vi "ATF RIg Graphs V1.1.vi"() -> ()   [LabVIEW 2022 SP3]
uses:
  Source code/Globals/ATF1_ACQ.vi
  Source code/Globals/Main_global.vi
panel:
  out "?":waveform(dbl)[](graph)
  out "?":cluster{dbl, dbl, dbl, dbl, dbl, dbl}(graph)
  out "?":waveform(dbl)[](graph)
  out "?":T1(graph)
  out "?":waveform(dbl)[](graph)
  out "?":cluster{dbl, dbl, dbl, dbl, "Drive_RPM":u32}(graph)
  # "Agnikul Cosmos Private Limited."
  # "ATF       Pump Rig Graph GUI     V1.0"
  # "MOTOR GRAPHS"
  # "PUMP GRAPHS"
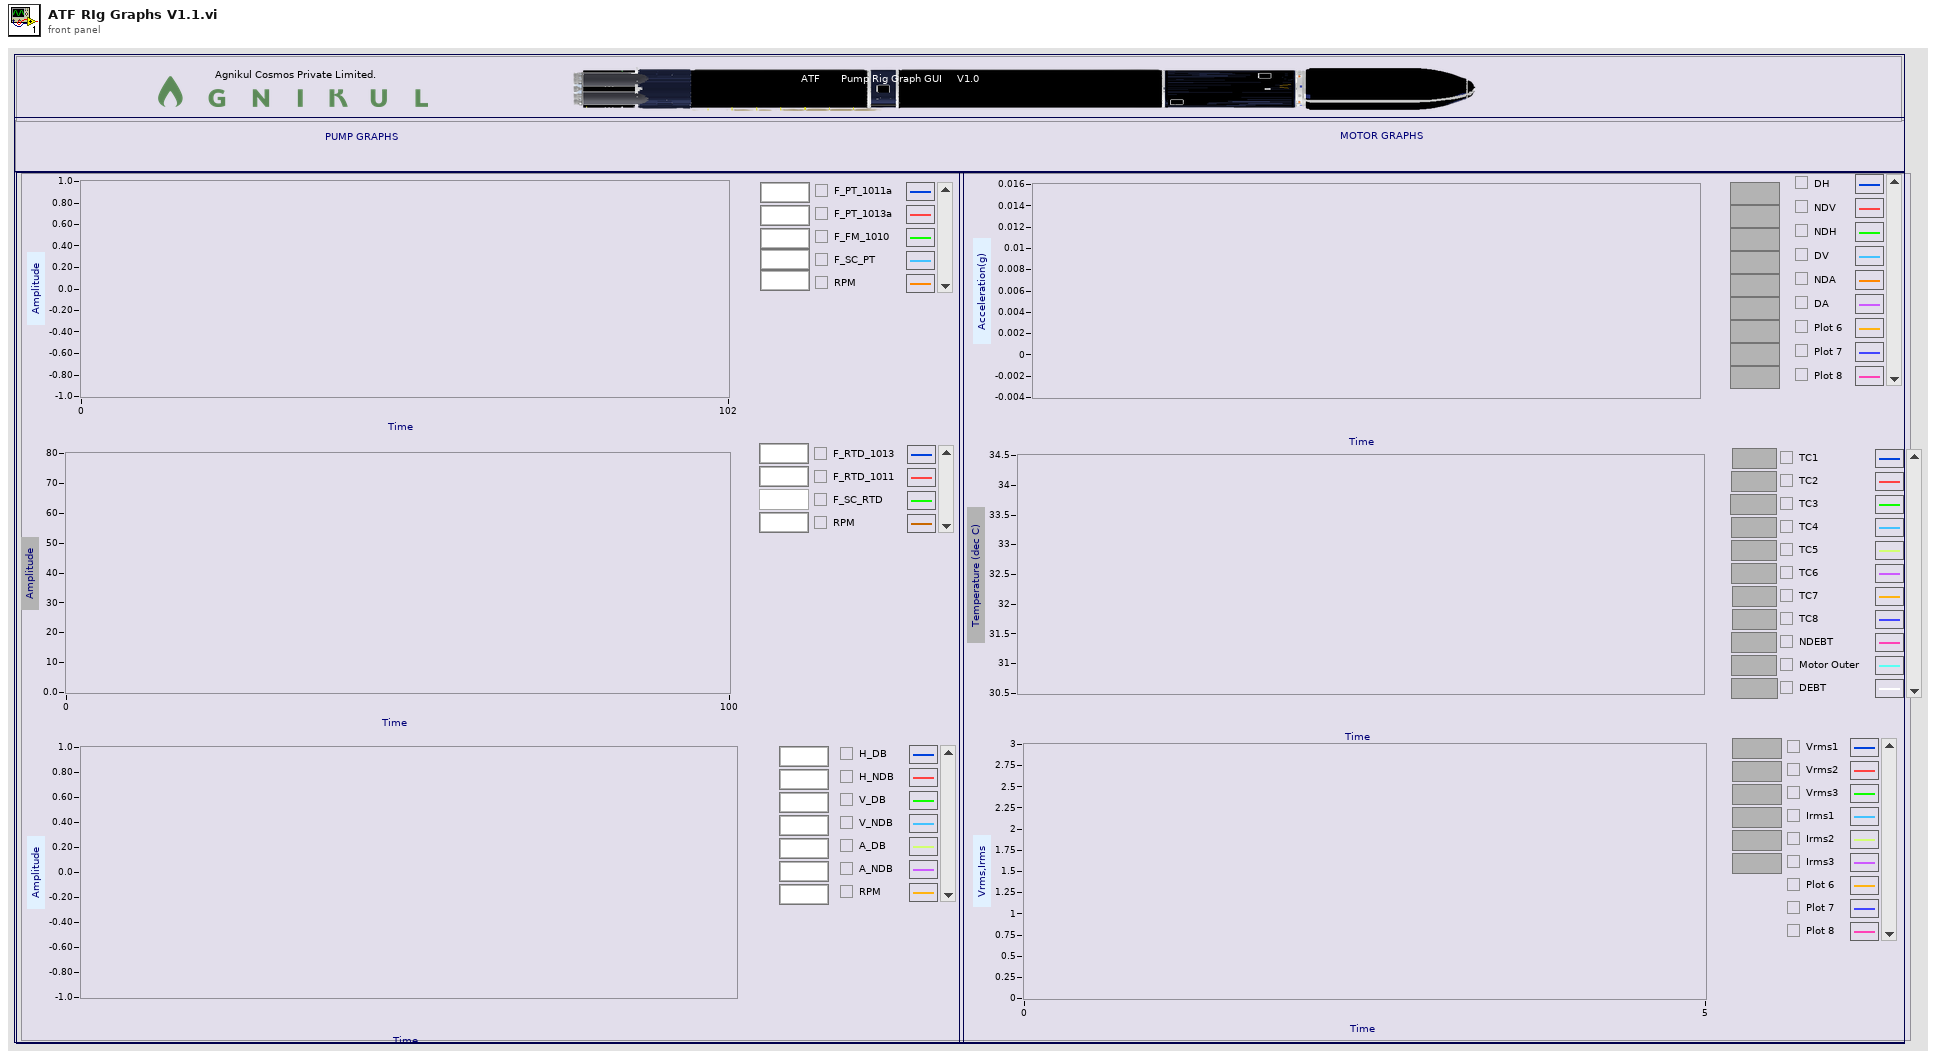
[diagram p1: front panel]
types:
  T1 = cluster{dbl, dbl, "element":dbl, "Drive_RPM":u32}
  T2 = cluster{dbl, "element":dbl, dbl, "Drive_RPM":u32}
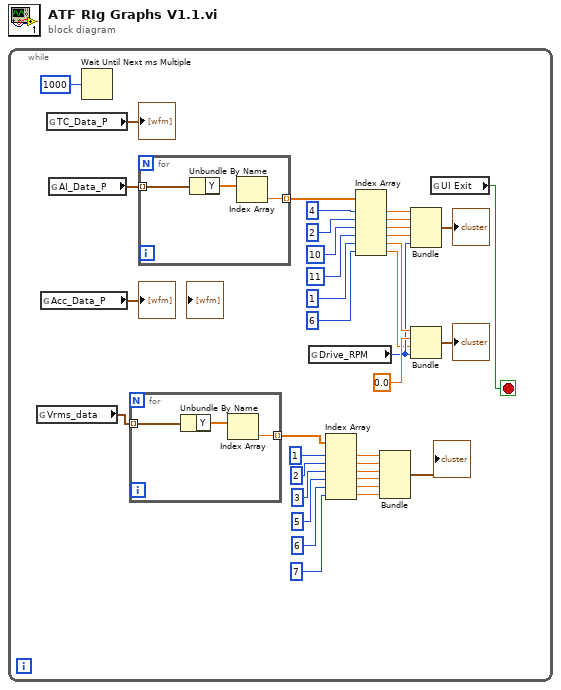
[diagram p0: block diagram]
diagram:
  n1 = while {
    stop <- w16 stop-if-true
    n2 = global read "ATF1_ACQ.vi" "Vrms_data"() -> (w15:waveform(dbl)[])
    n3 = global read "ATF1_ACQ.vi" "Acc_Data_P"() -> (→"?":waveform(dbl)[])
    n4 = global read "ATF1_ACQ.vi" "TC_Data_P"() -> (→"?":waveform(dbl)[])
    n5 = global read "ATF1_ACQ.vi" "AI_Data_P"() -> (w37:waveform(dbl)[])
    n6 = Wait Until Next ms Multiple(millisecond multiple=u32 1000) -> ()  [unwired: 1 out]
    n7 = for {
      tunnel: w15 -> [w40] mode=indexing
      tunnel: [w38] -> w14 mode=indexing
      n8 = Unbundle By Name(w40) -> ("Y"=w39:dbl[])
      n9 = Index Array(array=w39) -> (element=w38:dbl)  [unwired: 1 in]
    }
    n10 = for {
      tunnel: w37 -> [w43] mode=indexing
      tunnel: [w41] -> w36 mode=indexing
      n11 = Unbundle By Name(w43) -> ("Y"=w42:dbl[])
      n12 = Index Array(array=w42) -> (element=w41:dbl)  [unwired: 1 in]
    }
    n13 = global read "ATF1_ACQ.vi" "Drive_RPM"() -> (w21:u32)
    n14 = Index Array(array=w14, index #1=1 ("index"), index #2=2 ("index"), index #3=3 ("index"), index #4=5 ("index"), index #5=6 ("index"), index #6=7 ("index")) -> (element #1=w10:dbl, element #2=w9:dbl, element #3=w8:dbl, element #4=w3:dbl, element #5=w2:dbl, element #6=w1:dbl)
    n15 = Index Array(array=w36, index #1=4 ("index"), index #2=2 ("index"), index #3=10 ("index"), index #4=11 ("index"), index #5=1 ("index"), index #6=6 ("index")) -> (element #1=w27:dbl, element #2=w26:dbl, element #3=w25:dbl, element #4=w22:dbl, element #5=w24:dbl, element #6=w17:dbl)
    n16 = Bundle(w10, w9, w8, w3, w2, w1) -> (→"?":cluster{dbl, dbl, dbl, dbl, dbl, dbl})  [unwired: 1 in]
    n17 = Bundle(w27, w26, w25, w22, "Drive_RPM"=w21) -> (→"?":cluster{dbl, dbl, dbl, dbl, "Drive_RPM":u32})  [unwired: 1 in]
    n18 = Bundle(w24, "element"=0.0, w17, "Drive_RPM"=w21) -> (→"?":T2)  [unwired: 1 in]
    n19 = global read "Main_global.vi" "UI Exit"() -> (w16:bool)
  }
